vi "serial_data_parser.vi"() -> ()   [LabVIEW 2018]
panel:
  out "token index":i32
  out "appended array":dbl[](array[numeric])
  in  "input string":string
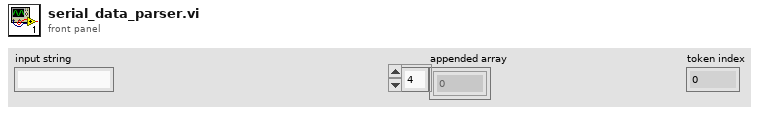
[diagram p1: front panel]
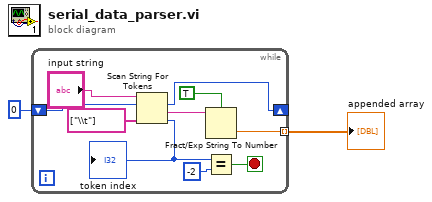
[diagram p0: block diagram]
diagram:
  n1 = while {
    shift-right: [w8] -> _
    shift-left: 0 ("offset past token") -> [w12]
    tunnel: [w5] -> w1 mode=indexing
    stop <- w3 stop-if-true
    n2 = Scan String For Tokens(6:string[] ["\\t"] ("delimiters (\\s,\\t,\\r,\\n)"), 8:w12, 9:"input string") -> (0:w10:i32, 1:w6:string, 2:w8:i32)  [unwired: 3 in, 1 out]
    "token index" <- w10
    n3 = Fract/Exp String To Number(use system decimal point (T)=TRUE, string=w6) -> (number=w5:dbl)  [unwired: 2 in, 1 out]
    n4 = Equal?(x=w10, y=-2) -> (x = y?=w3:bool)
  }
  "appended array" <- w1
